vi "MacroExecTest.vi"(8 "Error In":errorcluster, 11 "Macro IN":string[](array[string])) -> (0 "Error Out":errorcluster)   [LabVIEW 2012]
uses:
  Custom Controls and Typedefs/MacroExecutionStates.ctl
  Custom Controls and Typedefs/MacroConfirmationFlags.ctl
  <vilib>/regexp/Match Regular Expression.xnode
  GFG/GFG library.lvlib
panel:
  in  "Array 3":string[](array[string])=["LOOP.Start(iterations,2)", "Pause(wait.seconds,1)", "LOOP.Start(iterations,3)", "Pause(wait.seconds,2)", "LOOP.End", "LOOP.End", ""]
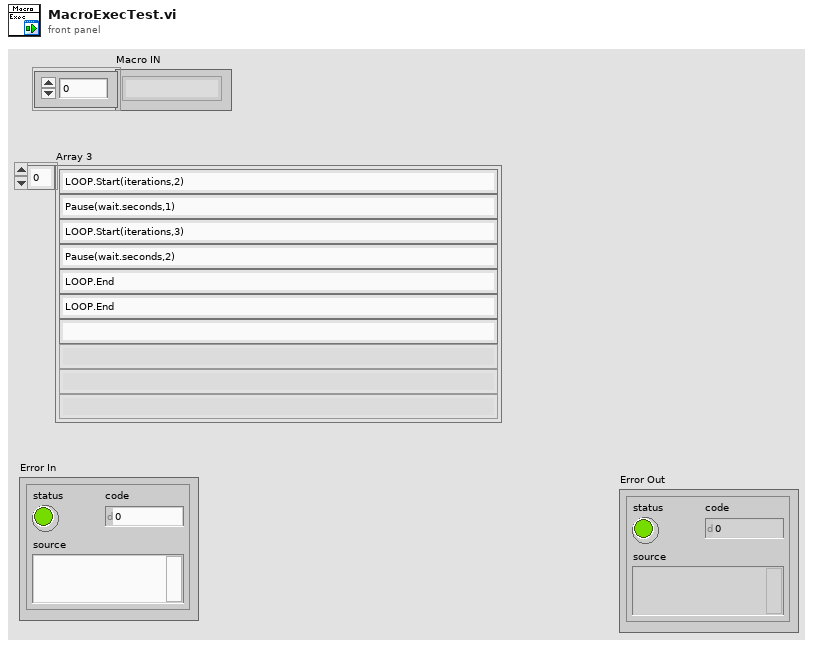
[diagram p1: front panel]
types:
  T1 = typedef "MacroExecutionStates.ctl" = enum16{"UI Mode", "Execute Command", "Wait for completion", "Pause"}
  T2 = typedef "MacroConfirmationFlags.ctl" = enum16{"None", "Flag_MovePos_Complete?", "Flag_Record_Complete?"}
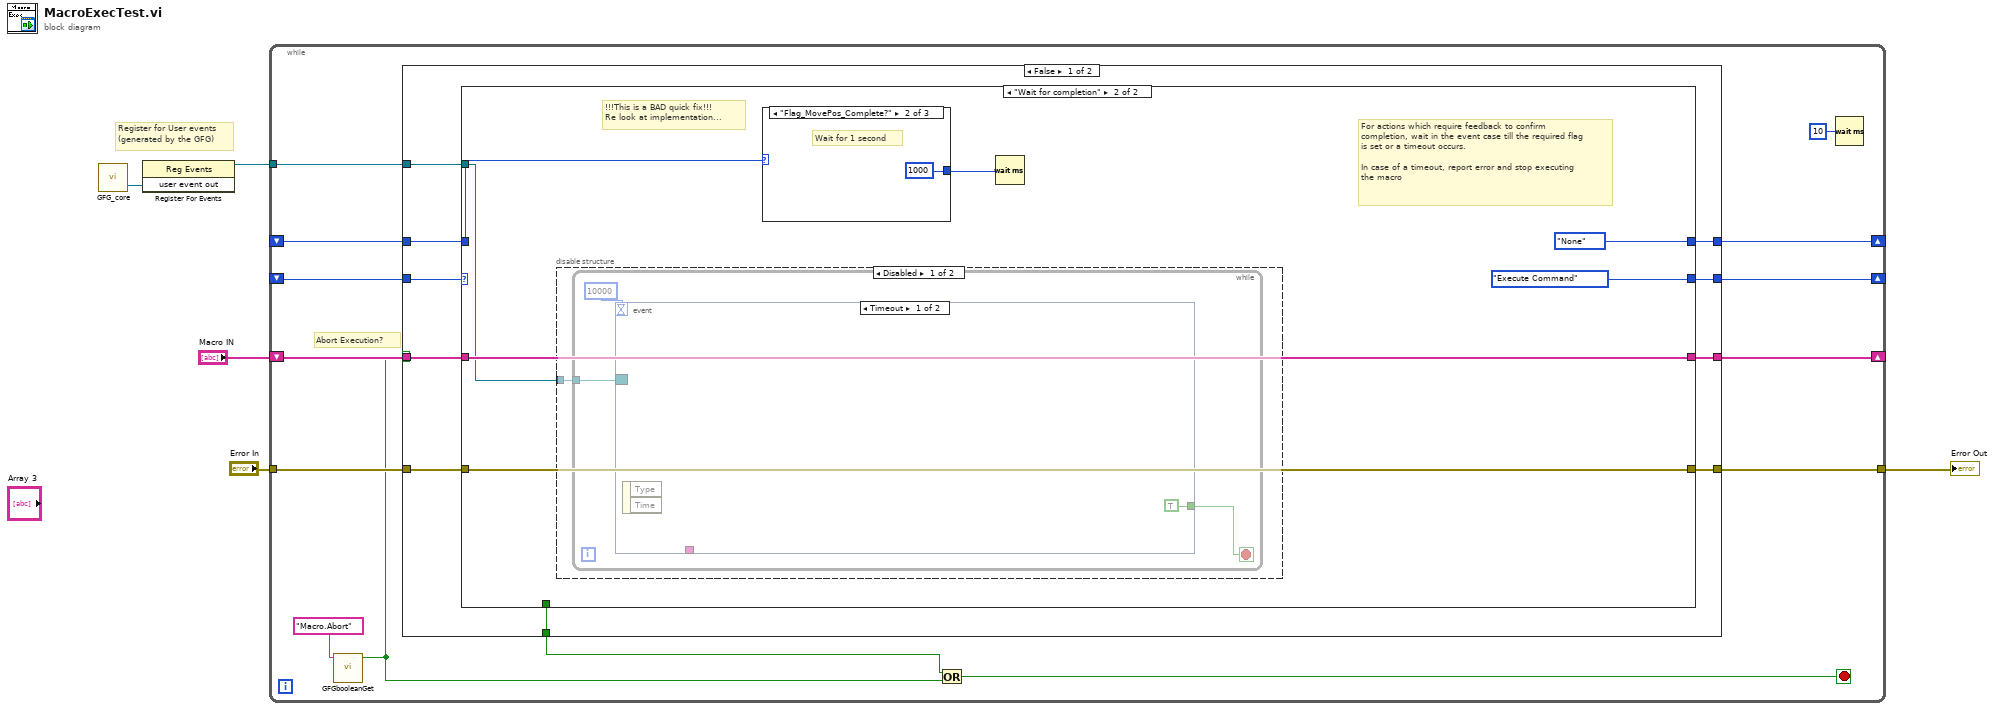
[diagram p0: block diagram]
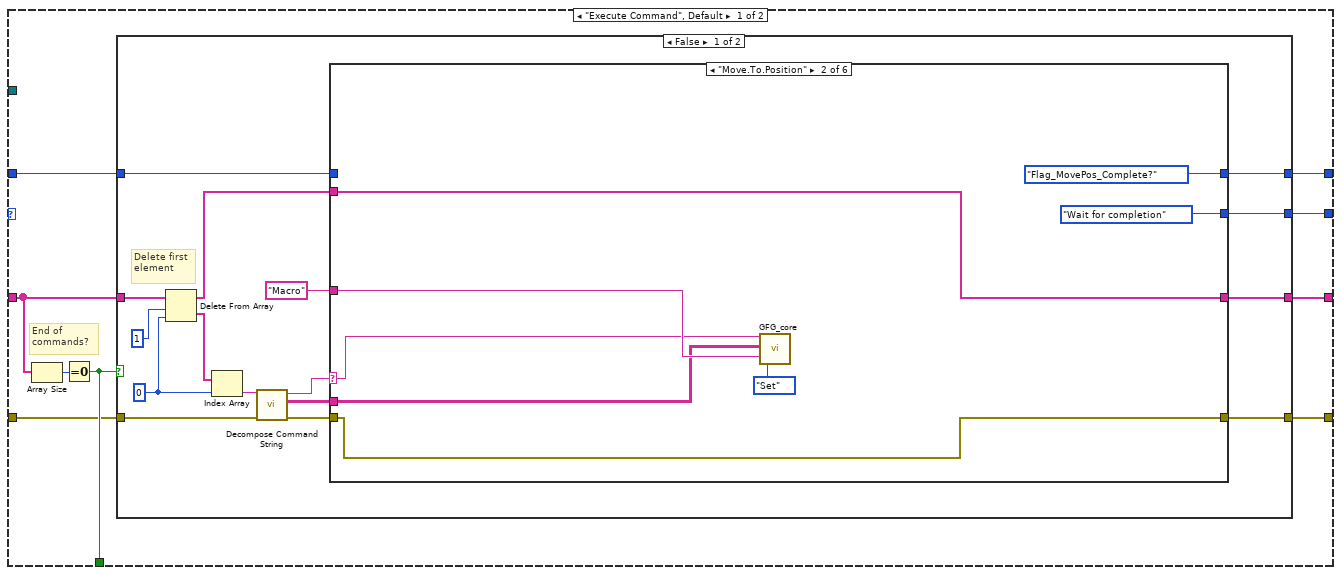
[diagram p2: hidden frame]
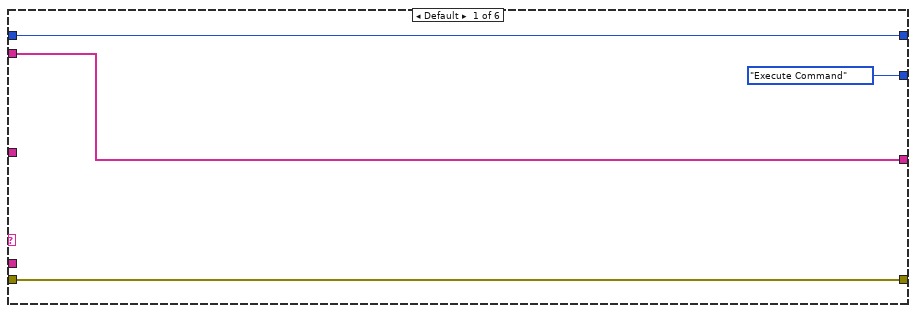
[diagram p3: hidden frame]
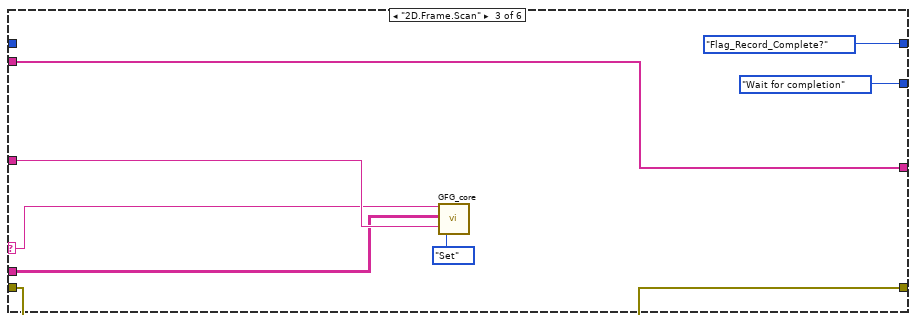
[diagram p4: hidden frame]
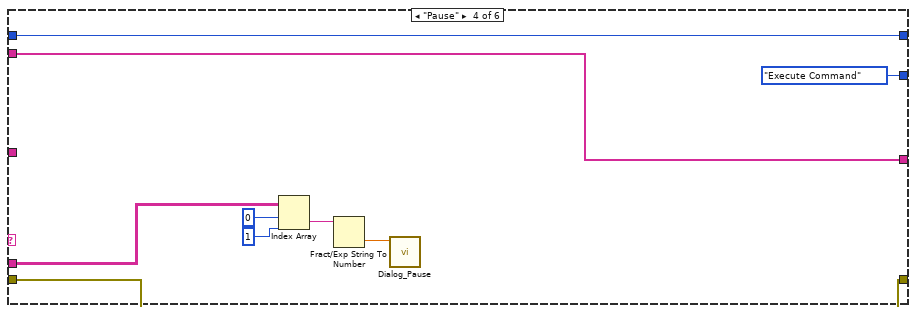
[diagram p5: hidden frame]
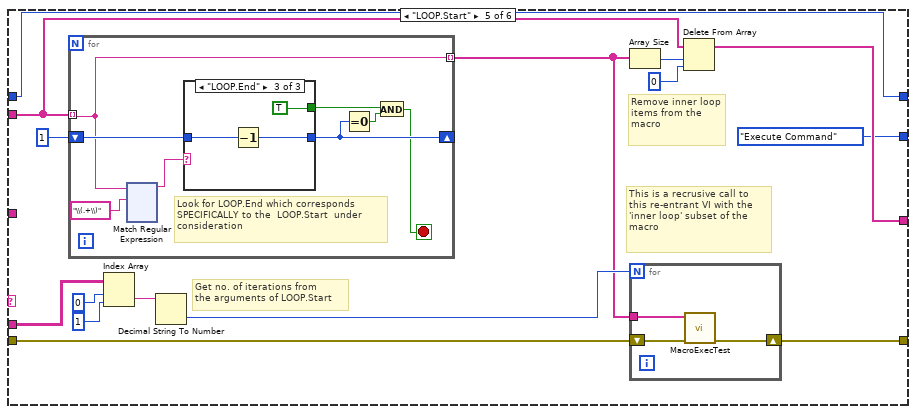
[diagram p6: hidden frame]
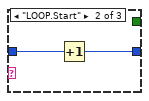
[diagram p8: hidden frame]
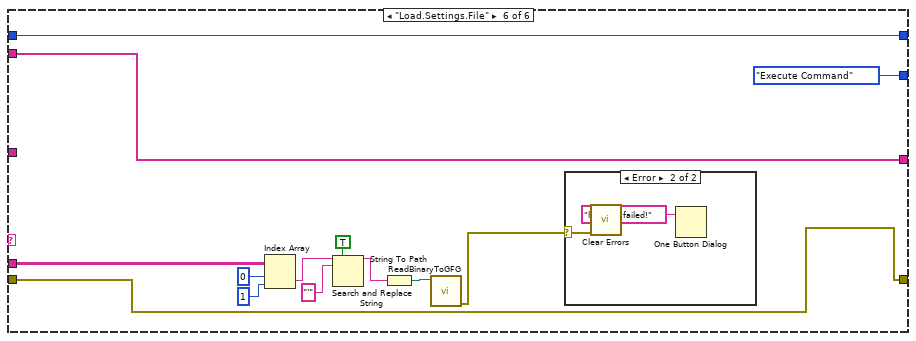
[diagram p9: hidden frame]
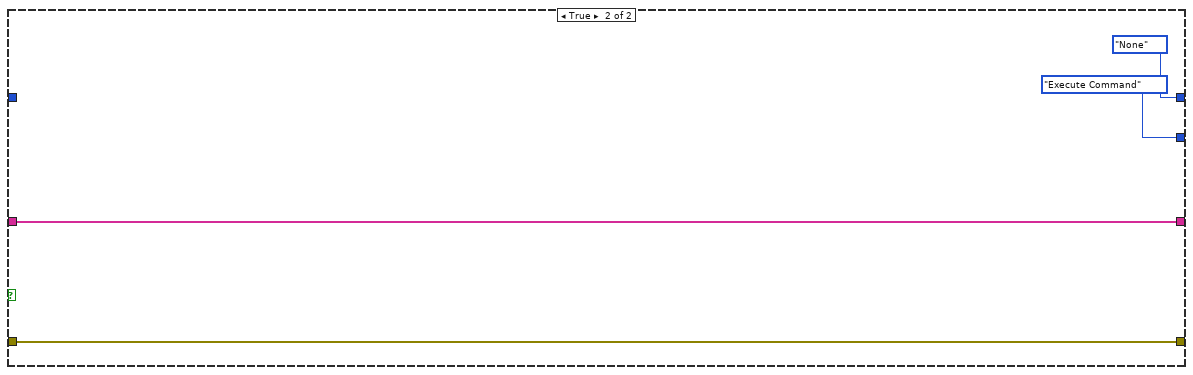
[diagram p11: hidden frame]
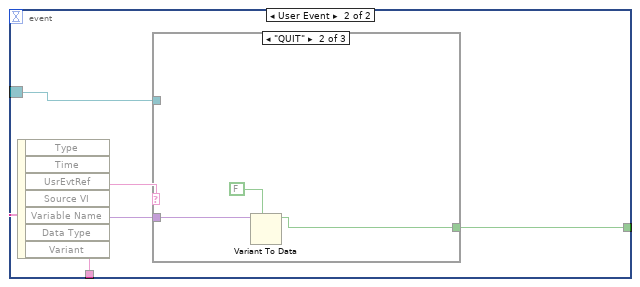
[diagram p12: hidden frame]
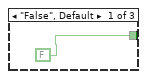
[diagram p13: hidden frame]
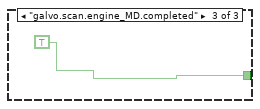
[diagram p14: hidden frame]
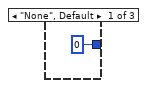
[diagram p16: hidden frame]
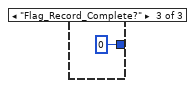
[diagram p17: hidden frame]
diagram:
  # "Register for User events\n(generated by the GFG)"
  n1 = call "GFG_core.vi"() -> ("user event out"=w1:refnum<user-event>)  [unwired: 13 in, 6 out]
  n2 = register-events(w1) -> (reference out=w2:refnum<event-registration>)  [unwired: 2 in, 1 out]
  n3 = while {
    shift-right: [w17] -> _
    shift-left: "Macro IN" -> [w19]
    tunnel: "Error In" -> [w18]
    tunnel: [w16] -> w4
    shift-right: [w14] -> _
    shift-left: _ -> [w12]
    shift-right: [w13] -> _
    shift-left: _ -> [w11]
    tunnel: w2 -> [w10]
    stop <- w7 stop-if-true
    # "Abort Execution?"
    n4 = call "GFGbooleanGet.vi"("Variable Name in"="Macro.Abort") -> ("Boolean"=w6:bool)  [unwired: 10 in]
    n5 = case shown="False" w6 {
      tunnel: w19 -> [w29 w271]
      tunnel: w18 -> [w28 w270]
      tunnel: [w27 w271] -> w17
      tunnel: [w26 w270] -> w16
      tunnel: [w25 w272] -> w14
      tunnel: [w24 w273] -> w13
      tunnel: w12 -> [w23 w272]
      tunnel: w11 -> [w22 w273]
      tunnel: w10 -> [w21 _]
      tunnel: [w20 _] -> w8
      frame False {
        n6 = case shown="\"Wait for completion\"" w23 {
          tunnel: w29 -> [w38 w252]
          tunnel: [w36 _] -> w20
          tunnel: w28 -> [w35 w251]
          tunnel: [w34 w252] -> w27
          tunnel: [w33 w251] -> w26
          tunnel: [w32 MacroExecutionStates."Execute Command" ("Macro Execution States")] -> w25
          tunnel: [w31 MacroConfirmationFlags."None" ("Macro Confirmation Flags")] -> w24
          tunnel: w22 -> [w30 w247]
          tunnel: w21 -> [_ w246]
          frame "Execute Command", Default {
            # "End of\ncommands?"
            n7 = Array Size(array=w38) -> (size(s)=w37:i32)
            n8 = Equal To 0?(x=w37) -> (x = 0?=w36:bool)
            n9 = case shown="False" w36 {
              tunnel: w38 -> [w51 w245]
              tunnel: w35 -> [w46 w244]
              tunnel: [w48 w245] -> w34
              tunnel: [w47 w244] -> w33
              tunnel: [w41 MacroExecutionStates."Execute Command" ("Macro Execution States")] -> w32
              tunnel: [w40 MacroConfirmationFlags."None" ("Macro Confirmation Flags")] -> w31
              tunnel: w30 -> [w39 _]
              frame False {
                w53 = 0 ("index")
                # "Delete first element"
                n10 = Delete From Array(array=w51, length=1, index=w53) -> (deleted portion=w52:string[], array with subset deleted=w49:string[])
                n11 = Index Array(array=w52, index=w53) -> (element=w42:string)
                n12 = call "Decompose Command String.vi"("Error In"=w46, "Command IN"=w42) -> ("Error Out"=w45:errorcluster, "ArgumentTable"=w43:string[][], "Action"=w44:string)  [unwired: 7 in]
                n13 = case shown="\"Move.To.Position\"" w44 {
                  selector: w44 -> [_ w60 w68 _ _ _]
                  tunnel: w43 -> [_ w59 w67 w82 w89 w237]
                  tunnel: "Macro" ("before match") -> [_ w61 w69 _ _ _]
                  tunnel: w49 -> [w58 w66 w74 w83 w95 w238]
                  tunnel: w45 -> [w57 w65 w73 w79 w97 w232]
                  tunnel: [w58 w66 w74 w83 w93 w238] -> w48
                  tunnel: [w57 w65 w73 w79 w92 w232] -> w47
                  tunnel: [MacroExecutionStates."Execute Command" ("Macro Execution States") MacroExecutionStates."Wait for completion" ("Macro Execution States") MacroExecutionStates."Wait for completion" ("Macro Execution States") MacroExecutionStates."Execute Command" ("Macro Execution States") MacroExecutionStates."Execute Command" ("Macro Execution States") MacroExecutionStates."Execute Command" ("Macro Execution States")] -> w41
                  tunnel: [w55 MacroConfirmationFlags."Flag_MovePos_Complete?" ("Macro Confirmation Flags") MacroConfirmationFlags."Flag_Record_Complete?" ("Macro Confirmation Flags") w75 w84 w227] -> w40
                  tunnel: w39 -> [w55 _ _ w75 w84 w227]
                  frame Default {
                  }
                  frame "Move.To.Position" {
                    n14 = call "GFG_core.vi"("Variable Name in"=w60, "Variant in"=w59, "Source VI"=w61, "Action"=enum16{"Init", "Set", "Get", "Clear"}."Set") -> ()  [unwired: 9 in, 7 out]
                  }
                  frame "2D.Frame.Scan" {
                    n15 = call "GFG_core.vi"("Variable Name in"=w68, "Variant in"=w67, "Source VI"=w69, "Action"=enum16{"Init", "Set", "Get", "Clear"}."Set") -> ()  [unwired: 9 in, 7 out]
                  }
                  frame "Pause" {
                    n16 = Index Array(array=w82, index (row)=0, index (col)=1 ("disabled index (col)")) -> (element=w78:string)
                    n17 = Fract/Exp String To Number(string=w78) -> (number=w77:dbl)  [unwired: 3 in, 1 out]
                    n18 = call "Dialog_Pause.vi"("Wait (s)"=w77) -> ()  [unwired: 11 in]
                  }
                  frame "LOOP.Start" {
                    # "This is a recrusive call to this re-entrant VI with the\n'inner loop' subset of the macro"
                    # "Remove inner loop items from the macro"
                    # "Get no. of iterations from\nthe arguments of LOOP.Start"
                    n19 = for {
                      tunnel: w95 -> [w99] mode=indexing
                      shift-right: [w105] -> _
                      shift-left: 1 ("length") -> [w106]
                      tunnel: [w99] -> w90 mode=indexing
                      stop <- w102 stop-if-true
                      # "Look for LOOP.End which corresponds\nSPECIFICALLY to the  LOOP.Start  under\nconsideration"
                      n20 = xnode "Match Regular Expression"("input string"=w99, "regular expression"="\\(.+\\)" ("search string/char (-)")) -> ("before match"=w100:string)  [unwired: 4 in, 4 out]
                      n21 = case shown="\"LOOP.End\"" w100 {
                        tunnel: w106 -> [w218 w220 w223]
                        tunnel: [w218 w219 w222] -> w105
                        tunnel: [_ _ TRUE] -> w103
                        frame Default {
                        }
                        frame "LOOP.Start" {
                          n22 = Increment(x=w220) -> (x+1=w219:i32)
                        }
                        frame "LOOP.End" {
                          n23 = Decrement(x=w223) -> (x-1=w222:i32)
                        }
                      }
                      n24 = Equal To 0?(x=w105) -> (x = 0?=w104:bool)
                      n25 = And(x=w103, y=w104) -> (x .and. y?=w102:bool)
                    }
                    n26 = Index Array(array=w89, index (row)=0, index (col)=1 ("disabled index (col)")) -> (element=w86:string)
                    n27 = Decimal String To Number(string=w86) -> (number=w98:i32)  [unwired: 2 in, 1 out]
                    n28 = Array Size(array=w90) -> (size(s)=w94:i32)
                    n29 = for {
                      N: w98 -> [_]
                      shift-right: [w225] -> w92
                      shift-left: w97 -> [w226]
                      tunnel: w90 -> [w224]
                      n30 = call "MacroExecTest.vi"("Error In"=w226, "Macro IN"=w224) -> ("Error Out"=w225:errorcluster)  [unwired: 9 in]
                    }
                    n31 = Delete From Array(array=w95, length=w94, index=0) -> (array with subset deleted=w93:string[])  [unwired: 1 out]
                  }
                  frame "Load.Settings.File" {
                    n32 = Index Array(array=w237, index (row)=0, index (col)=1 ("index")) -> (element=w230:string)
                    n33 = Search and Replace String(replace all?=TRUE ("replace all? (F)"), input string=w230, search string="'") -> (result string=w228:string)  [unwired: 5 in, 3 out]
                    n34 = String To Path(string=w228) -> (path=w239:path)
                    n35 = call "ReadBinaryToGFG.vi"("file path"=w239) -> ("error IO"=w233:errorcluster)  [unwired: 10 in]
                    n36 = case shown="Error" w233 {
                      selector: w233 -> [_ w241]
                      frame No Error {
                      }
                      frame Error {
                        n37 = call <vilib>:"Clear Errors.vi"("error in (no error)"=w241) -> ()  [unwired: 6 in, 1 out]
                        n38 = One Button Dialog(message="load file failed!") -> ()  [unwired: 1 in, 1 out]
                      }
                    }
                  }
                }
              }
              frame True {
              }
            }
          }
          frame "Wait for completion" {
            # "!!!This is a BAD quick fix!!! \nRe look at implementation..."
            # "For actions which require feedback to confirm completion, wait in the event case till the required flag is set or a timeout occurs.\n\nIn case of a timeout, report error and stop executing the macro"
            n39 = disable-structure shown="Disabled" {
              disable-tunnel: w246 -> [w253 _]
              frame Disabled {
                n40 = while {
                  tunnel: w253 -> [w256]
                  stop <- w255 stop-if-true
                  n41 = event shown="[0] Timeout" {
                    selector: w256 -> [_ w259]
                    dyn-events: _ -> [_ _]
                    timeout: 10000 -> [_ _]
                    tunnel: [_ w260] -> _
                    tunnel: [TRUE ("NewVal") w258] -> w255
                    event Timeout {
                      n42 = event-data() -> ()  [unwired: 1 in, 2 out]
                    }
                    event User Event {
                      n43 = event-data() -> ("Variable Name"=w260:string, "Variant"=w261:variant)  [unwired: 1 in, 5 out]
                      n44 = case shown="\"QUIT\"" w260 {
                        tunnel: [FALSE ("NewVal") w263 TRUE ("NewVal")] -> w258
                        tunnel: w261 -> [_ w265 _]
                        tunnel: w259 -> [_ _ _]
                        frame "False", Default {
                        }
                        frame "QUIT" {
                          n45 = Variant To Data(type=FALSE ("NewVal"), Variant=w265) -> (data=w263:bool)  [unwired: 1 in, 1 out]
                        }
                        frame "galvo.scan.engine_MD.completed" {
                        }
                      }
                    }
                  }
                }
              }
              frame Enabled {
              }
            }
            n46 = case shown="\"Flag_MovePos_Complete?\"" w247 {
              tunnel: [u32 0 ("milliseconds to wait") u32 1000 ("milliseconds to wait") u32 0 ("milliseconds to wait")] -> w248
              frame "None", Default {
              }
              frame "Flag_MovePos_Complete?" {
                # "Wait for 1 second"
              }
              frame "Flag_Record_Complete?" {
              }
            }
            n47 = Wait (ms)(milliseconds to wait=w248) -> ()  [unwired: 1 out]
          }
        }
      }
      frame True {
      }
    }
    n48 = Or(x=w8, y=w6) -> (x .or. y?=w7:bool)
    n49 = Wait (ms)(milliseconds to wait=u32 10) -> ()  [unwired: 1 out]
  }
  "Error Out" <- w4
